vi "4PtsPointFunction.vi"(8 "4PointB":cluster{sgl, sgl}[][](array[cluster]), 9 "4PointA":cluster{"[0]":sgl, "[1]":sgl}[][](array[cluster]), 10 "PointIn":cluster{"X":dbl, "Y":dbl}, 11 "Index":cluster{i32, i32}) -> (3 "PointOut":cluster{"OX":dbl, "OY":dbl})   [LabVIEW 2012]
panel:
  out "subarray":dbl[](array[numeric])
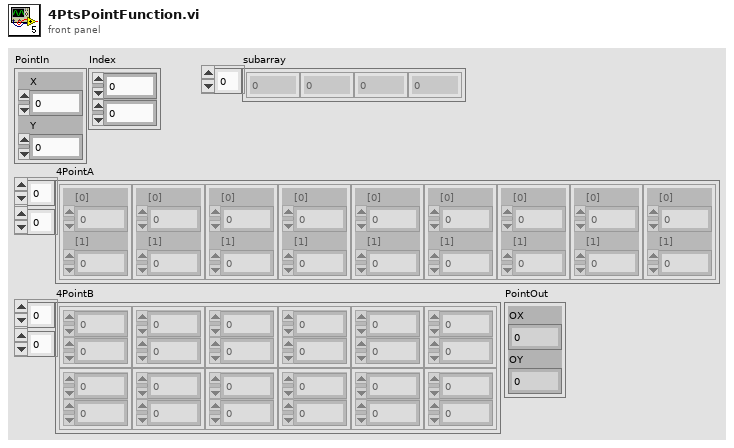
[diagram p1: front panel]
types:
  T1 = typedef "NI_Matrix.lvlib/RealMatrix.ctl" = dbl[][]
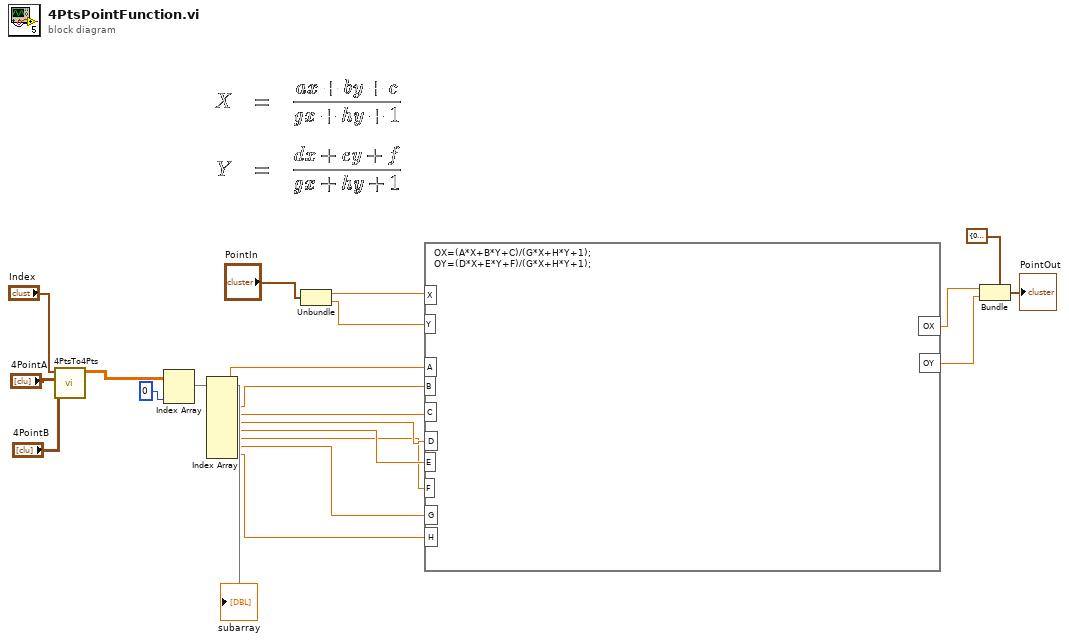
[diagram p0: block diagram]
diagram:
  n1 = call "4PtsTo4Pts.vi"("4PointB"="4PointB", "4PointA"="4PointA", "index"="Index") -> ("A x B"=w21:T1)  [unwired: 8 in]
  n2 = Index Array(array=w21, index (col)=0 ("index (row)")) -> (element=w20:dbl[])  [unwired: 1 in]
  "subarray" <- w20
  n3 = Index Array(array=w20) -> (element #1=w19:dbl, element #2=w18:dbl, element #3=w17:dbl, element #4=w16:dbl, element #5=w15:dbl, element #6=w14:dbl, element #7=w13:dbl, element #8=w12:dbl)  [unwired: 8 in]
  n4 = Unbundle("PointIn") -> ("X"=w10:dbl, "Y"=w9:dbl)
  n5 = formula code="OX=(A*X+B*Y+C)/(G*X+H*Y+1);\nOY=(D*X+E*Y+F)/(G*X+H*Y+1);"("X"=w10, "Y"=w9, "A"=w19, "B"=w18, "C"=w17, "D"=w16, "E"=w15, "F"=w14, "G"=w13, "H"=w12) -> ("OY"=w4:dbl, "OX"=w5:dbl)
  n6 = Bundle(cluster=cluster{"OX":dbl, "OY":dbl} {"OX"=0.0, "OY"=0.0}, "OX"=w5, "OY"=w4) -> (→"PointOut":cluster{"OX":dbl, "OY":dbl})
